vi "LQR_CLEst.vi"() -> ()   [LabVIEW 2019]
uses:
  <vilib>/Analysis/Matrix/Datatypes/RealMatrix.ctl
  <vilib>/Platform/TimedLoop/XDataNode/timing_clust.ctl
  <vilib>/Platform/TimedLoop/XDataNode/nitl_modes.ctl
  <vilib>/Platform/TimedLoop/XDataNode/wakeup.ctl
  <vilib>/Simulation/Shared/_Datatypes/SIM SISO Transfer Function.ctl
  <vilib>/myRIO/Instrument Drivers/Onboard IO/AI/typedefs/AI Reference.ctl
  <vilib>/myRIO/Common/Instrument Driver Framework/Utilities/typedefs/myRIO Generic Hardware Reference.ctl
  <vilib>/myRIO/Common/Instrument Driver Framework/Utilities/typedefs/Hardware Version Enum.ctl
  <vilib>/myRIO/Common/Instrument Driver Framework/Utilities/typedefs/myRIO v1.0 Reference.ctl
  <vilib>/myRIO/Common/Instrument Driver Framework/Utilities/typedefs/Generic FPGA Reference.ctl
  <vilib>/myRIO/Common/Instrument Driver Framework/myRIO v1.0/AI/typedefs/AI Channels List.ctl
  <vilib>/myRIO/Common/Instrument Driver Framework/myRIO v1.0/AI/typedefs/AI Channels Enum.ctl
  <vilib>/myRIO/Common/Instrument Driver Framework/Utilities/typedefs/Analog Scaling Constants List.ctl
  <vilib>/myRIO/Common/Instrument Driver Framework/Utilities/typedefs/Analog Scaling Constants.ctl
  <vilib>/userDefined/High Color/nirio_resource_hc.ctl
  <vilib>/myRIO/Instrument Drivers/Onboard IO/AO/typedefs/AO Reference.ctl
  <vilib>/myRIO/Common/Instrument Driver Framework/myRIO v1.0/AO/typedefs/AO Channels List.ctl
  <vilib>/myRIO/Common/Instrument Driver Framework/myRIO v1.0/AO/typedefs/AO Channels Enum.ctl
  <vilib>/myRIO/Common/Instrument Driver Framework/Utilities/vis/Is FPGA Ref Available.vi
  <vilib>/myRIO/Common/Instrument Driver Framework/myRIO v1.0/AI/vis/myRIO v1.1 Open AI.vi
  <vilib>/myRIO/Instrument Drivers/Onboard IO/AI/vis/Read.vi
  <vilib>/Simulation/DiscreteLinear/Implementation/NILVSim Discrete Transfer Function Direct.llb/SIM Discrete Transfer Function Diagram (SISO).vi
  <vilib>/myRIO/Common/Instrument Driver Framework/myRIO v1.0/AO/vis/myRIO v1.1 Open AO.vi
  <vilib>/myRIO/Instrument Drivers/Onboard IO/AO/vis/Write.vi
  <vilib>/myRIO/Common/Instrument Driver Framework/Utilities/vis/Validate Channels.vi
  <vilib>/myRIO/Common/Instrument Driver Framework/myRIO v1.0/AI/vis/myRIO v1.0 Reserve AI.vi
  <vilib>/Simulation/ContinuousLinear/Implementation/Shared/SIM Transfer Function Support.llb/SIM TransferFunction Normalize to Buffer.vi
  <vilib>/Simulation/DiscreteLinear/Implementation/Shared/SIM Init Discrete States.vi
  <vilib>/Simulation/DiscreteLinear/Implementation/NILVSim Discrete Transfer Function Direct.llb/SIM Transfer Function Direct core (SISO).vi
  <vilib>/myRIO/Common/Instrument Driver Framework/myRIO v1.0/AO/vis/myRIO v1.0 Reserve AO.vi
  <vilib>/myRIO/Common/Instrument Driver Framework/myRIO v1.0/AI/vis/myRIO v1.0 Build MUX Configuration AI.vi
  <vilib>/myRIO/Common/Instrument Driver Framework/myRIO v1.0/Resource Manager/vis/myRIO v1.0 Reserve Channel List.vi
  <vilib>/Simulation/ContinuousLinear/Implementation/Shared/SIM Transfer Function Support.llb/SIM TransferFunction Normalize.vi
  <vilib>/myRIO/Common/Instrument Driver Framework/myRIO v1.0/AO/vis/myRIO v1.0 Build MUX Configuration AO.vi
  <vilib>/myRIO/Common/Instrument Driver Framework/myRIO v1.0/Resource Manager/vis/myRIO v1.0 Reserve Channel.vi
  <vilib>/myRIO/Common/Instrument Driver Framework/myRIO v1.0/Resource Manager/vis/myRIO v1.0 Unreserve Channel.vi
  <vilib>/Simulation/Implementation/Shared/SIM Polynomials.llb/SIM Remove Zero Coefficients (DBL).vi
  <vilib>/myRIO/Common/Instrument Driver Framework/myRIO v1.0/Resource Manager/vis/myRIO v1.0 Build Mutex Name.vi
  <vilib>/Simulation/Implementation/Shared/SIM Polynomials.llb/SIM Divide Polynomials (DBL).vi
  <vilib>/Simulation/Implementation/Shared/SIM BuildSimErr.vi
  <vilib>/Utility/VariantDataType/GetNumericInfo.vi
  <vilib>/Utility/error.llb/Error Cluster From Error Code.vi
  <vilib>/myRIO/Common/Instrument Driver Framework/myRIO v1.0/myRIO v1.1 Open.vi
  <vilib>/myRIO/Common/Instrument Driver Framework/myRIO v1.0/AI/vis/myRIO v1.0 Get Scaling Constants AI.vi
  <vilib>/myRIO/Common/Instrument Driver Framework/Utilities/vis/IO Manager.vi
  <vilib>/myRIO/Common/Instrument Driver Framework/Utilities/vis/Configuration Manager.vi
  <vilib>/myRIO/Common/Instrument Driver Framework/myRIO v1.0/myRIO v1.0 Close.vi
  <vilib>/myRIO/Common/Instrument Driver Framework/myRIO v1.0/AI/vis/myRIO v1.0 Read AI.vi
  <vilib>/Analysis/Matrix/Numeric/Multiply/Multiply - RM,RM.vi
  <vilib>/Analysis/Matrix/Numeric/Subtract/Subtract (Elementwise) - R,RM.vi
  <vilib>/Analysis/Matrix/Numeric/Add/Add - RM,RM.vi
  <vilib>/myRIO/Common/Instrument Driver Framework/myRIO v1.0/AO/vis/myRIO v1.0 Get Scaling Constants AO.vi
  <vilib>/myRIO/Common/Instrument Driver Framework/myRIO v1.0/AO/vis/myRIO v1.0 Write AO.vi
  <vilib>/platform/TimedLoop/XDataNode/XDataNode.xnode
  <vilib>/Simulation/Implementation/XNodeFramework/SimXNode/SimX.xnode
  <vilib>/myRIO/Express VI/Onboard IO/AI/AI Express VI.xnode
  <vilib>/myRIO/Instrument Drivers/Onboard IO/AI/vis/myRIO AI Open.xnode
  <vilib>/myRIO/Express VI/Onboard IO/AO/AO Express VI.xnode
  <vilib>/myRIO/Instrument Drivers/Onboard IO/AO/vis/myRIO AO Open.xnode
  <vilib>/Analysis/Matrix/Numeric/Multiply/Multiply - RM,R.vi
  <vilib>/Platform/TimedLoop/XDataNode/XDNodeRunTimeDep.lvlib
  <vilib>/myRIO/Instrument Drivers/Onboard IO/AI/AI.lvlib
  <vilib>/myRIO/Instrument Drivers/Onboard IO/AO/AO.lvlib
  <vilib>/Analysis/Matrix/NI_Matrix.lvlib
panel:
  in  "amplitude":dbl=1.0 format="%0.2f"
  out "output y(k)":dbl=6.43996164946016e-05
  in  "D":dbl=7.3
  in  "P":dbl=5291.0
  out "x*y":dbl(graph)=-8.32082689025263
  in  "C":T1=[[1.0, 0.0]]
  out "transposed matrix":T1=[[7.6247197208905344e-06], [0.00010412510161981911]]
  in  "B":T1=[[0.0], [17.2685]]
  in  "A":T1=[[0.0, 1.0], [-5529.8, -0.5327]]
  in  "L":T1=[[2200.0], [1953300.0]]
  out "Iteration Duration":i64(graph)=347
  in  "esc":bool
  out "x[um]":cluster{dbl, dbl, dbl, dbl, "output y(k)":dbl}(graph)
  out "Current Output EM":dbl(graph)=0.03990822535355048
  in  "Stop EM + FRF":bool=TRUE
  out "left[V]":dbl=-0.0
  out "right[V]":dbl=-0.0
  out "um":dbl=376.9531636
  # "mA"
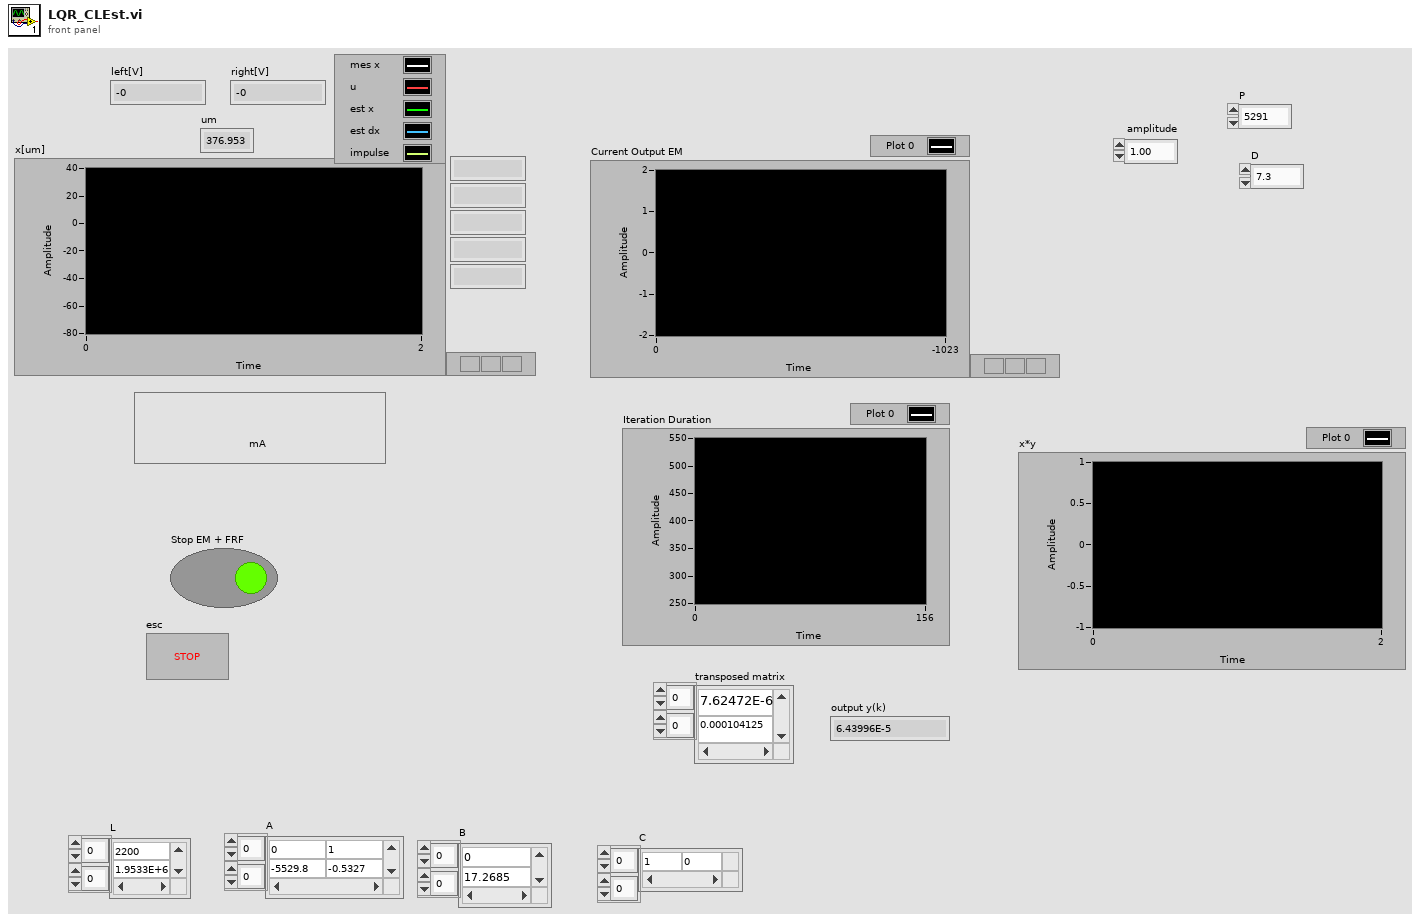
[diagram p1: front panel]
types:
  T1 = typedef "NI_Matrix.lvlib/RealMatrix.ctl" = dbl[][]
  T2 = typedef "XDNodeRunTimeDep.lvlib/timing_clust.ctl" = cluster{"Expected End [f-1]":u64, "Actual End [f-1]":u64, "Finished Late? [f-1]":bool, "Expected End [i-1]":u64, "Actual End [i-1]":u64, "Finished Late? [i-1]":bool, "Expected Start [i]":u64, "Actual Start [i]":u64, "Expected Start [f]":u64, "Actual Start [f]":u64, "Source Name":string, "Structure Name":string, "Period":i64, "Deadline":i64, "Offset":i64, "Start":i64, "Priority":i32, "Timeout":i32, "Mode":T3, "Wakeup Reason":T4, "Error":errorcluster, "Source Type":string, "Secondary Source Type":string, "Global End Time":u64, "Global Start Time":u64, "Frame Duration":u64, "Iteration Duration":u64, "Assigned CPU":i32, "I/O Scan Engine Mode":u32}
  T3 = typedef "XDNodeRunTimeDep.lvlib/nitl_modes.ctl" = enum32{"No Change", "Process missed periods, maintain original phase", "Discard missed periods, maintain original phase", "Process missed periods, ignore original phase", "Discard missed periods, ignore original phase"}
  T4 = typedef "XDNodeRunTimeDep.lvlib/wakeup.ctl" = enum32{"Normal", "Aborted", "Asynchronous wakeup", "Timing source error", "Timed loop error", "Timeout"}
  T5 = typedef "SIM SISO Transfer Function.ctl" = cluster{"Numerator":dbl[], "Denominator":dbl[]}
  T6 = typedef "AO.lvlib/AO Reference.ctl" = cluster{"myRIO Reference":T7, "AO Channel List":T11, "AO Scaling Constant List":T13}
  T7 = typedef "myRIO Generic Hardware Reference.ctl" = cluster{"myRIO Model":T8, "myRIO Hardware Reference":T9}
  T8 = typedef "Hardware Version Enum.ctl" = enum16{"Unknown", "myRIO-1900", "myRIO-1950", "roboRIO", "NI ELVIS RIO CM", "ELVIS III"}
  T9 = typedef "myRIO v1.0 Reference.ctl" = cluster{"Generic FPGA Reference":T10, "Allow multiple opens":bool}
  T10 = typedef "Generic FPGA Reference.ctl" = refnum<k20>
  T11 = typedef "AO Channels List.ctl" = T12[]
  T12 = typedef "AO Channels Enum.ctl" = enum16{"Not Connected", "AudioOut/Left", "AudioOut/Right", "C/AO0", "C/AO1", "A/AO0", "A/AO1", "B/AO0", "B/AO1"}
  T13 = typedef "Analog Scaling Constants List.ctl" = T14[]
  T14 = typedef "Analog Scaling Constants.ctl" = cluster{"LSB Weight (Volts)":dbl, "Offset (Volts)":dbl, "Signed?":bool}
  T15 = typedef "nirio_resource_hc.ctl" = tag
  T16 = typedef "AI.lvlib/AI Reference.ctl" = cluster{"myRIO Reference":T7, "AI Channels List":T17, "AI Scaling Constants List":T13}
  T17 = typedef "AI Channels List.ctl" = T18[]
  T18 = typedef "AI Channels Enum.ctl" = enum16{"Not Connected", "AudioIn/Left", "AudioIn/Right", "C/AI0", "C/AI1", "A/AI0", "A/AI1", "A/AI2", "A/AI3", "A/AI4", "A/AI5", "A/AI6", "A/AI7", "B/AI0", "B/AI1", "B/AI2", "B/AI3", "B/AI4", "B/AI5", "B/AI6", "B/AI7", "AI/AI0", "AI/AI1", "AI/AI2", "AI/AI3", "A/AI0 (DIFF)", "A/AI1 (DIFF)", "A/AI2 (DIFF)", "A/AI3 (DIFF)", "B/AI0 (DIFF)", "B/AI1 (DIFF)", "B/AI2 (DIFF)", "B/AI3 (DIFF)"}
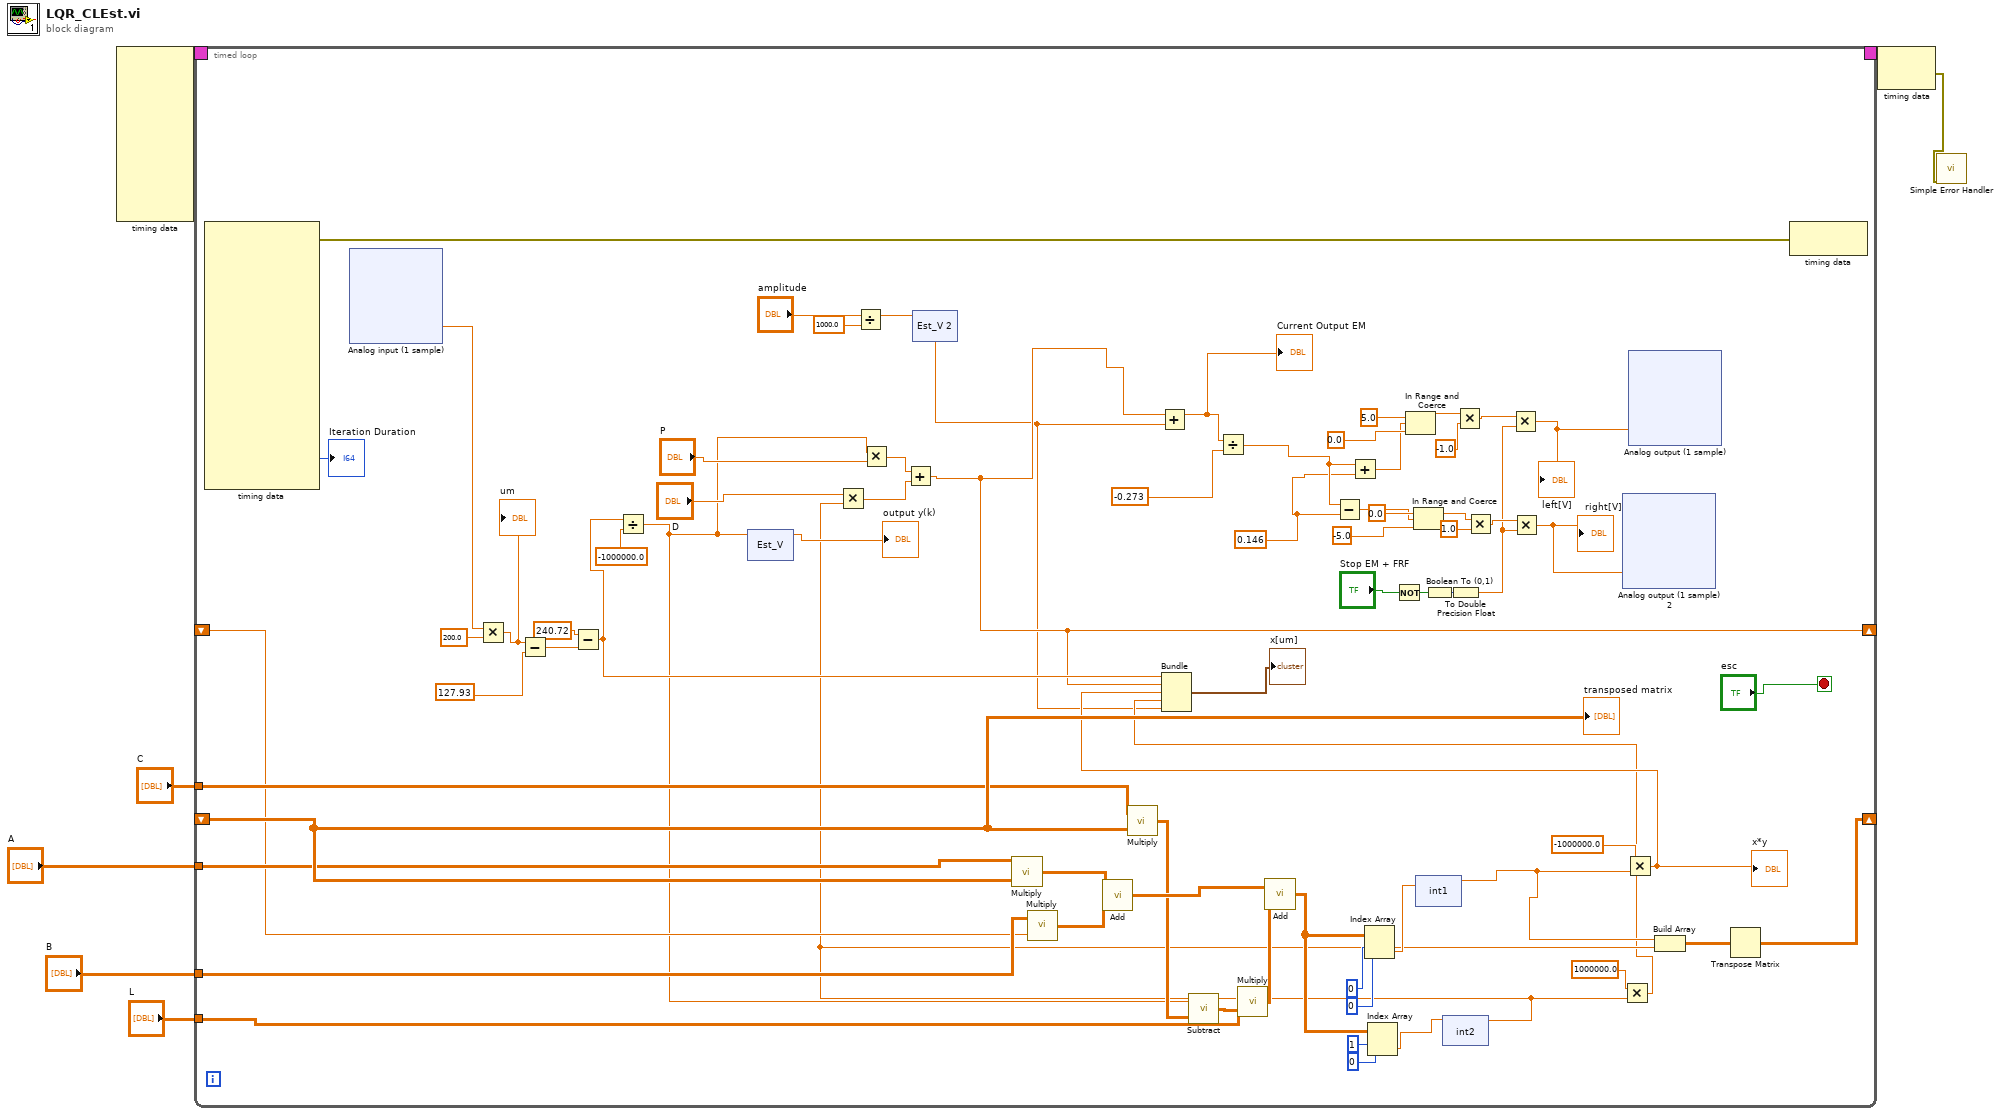
[diagram p0: block diagram]
diagram:
  n1 = node-c288() -> (w7:T2)  [unwired: 10 in]
  n2 = timed-loop {
    timing: w7 -> [_]
    timing-out: [_] -> w6
    shift-right: [w34] -> _
    shift-left: _ -> [w35]
    tunnel: "A" -> [w31]
    tunnel: "B" -> [w30]
    tunnel: "C" -> [w29]
    tunnel: "L" -> [w28]
    shift-right: [w9] -> _
    shift-left: _ -> [w25]
    stop <- "esc" stop-if-true
    w57 = 0.146 ("y")
    n3 = node-c288() -> (w79:errorcluster, →"Iteration Duration":i64)  [unwired: 1 in, 15 out]
    n4 = xnode "Analog input (1 sample)"() -> ("C/AI1 (AI1)"=w53:dbl)  [unwired: 1 in, 1 out]
    n5 = Multiply(x=w53, y=200.0) -> (x*y=w77:dbl)
    "um" <- w77
    n6 = Subtract(x=w77, y=127.93) -> (x-y=w76:dbl)
    n7 = Subtract(x=240.72, y=w76) -> (x-y=w47:dbl)
    n8 = Divide(x=w47, y=-1000000.0) -> (x/y=w18:dbl)
    n9 = xnode "Est_V"("input u(k)"=w18) -> ("output y(k)"=→"output y(k)":dbl)  [unwired: 2 in, 1 out]
    n10 = Divide(x="amplitude", y=1000.0) -> (x/y=w16:dbl)
    n11 = Multiply(x=w18, y="P") -> (x*y=w27:dbl)
    n12 = xnode "Est_V 2"("input u(k)"=w16) -> ("output y(k)"=w8:dbl)  [unwired: 2 in, 1 out]
    n13 = call-poly <vilib>:"Multiply.vi"("Real Matrix B"=w35, "Real Matrix A"=w31) -> ("A * B"=w46:T1)
    n14 = call-poly <vilib>:"Multiply.vi"("Real Scalar c"=w25, "Real Matrix A"=w30) -> ("A * c"=w45:T1)
    n15 = call-poly <vilib>:"Add.vi"("Real Matrix B"=w45, "Real Matrix A"=w46) -> ("A + B"=w44:T1)
    n16 = call-poly <vilib>:"Multiply.vi"("Real Matrix B"=w35, "Real Matrix A"=w29) -> ("A * B"=w33:T1)
    n17 = call-poly <vilib>:"Subtract.vi"("Real Matrix A"=w33, "Real Scalar c"=w18) -> ("c - A"=w37:T1)
    n18 = call-poly <vilib>:"Multiply.vi"("Real Matrix B"=w37, "Real Matrix A"=w28) -> ("A * B"=w43:T1)
    n19 = call-poly <vilib>:"Add.vi"("Real Matrix B"=w43, "Real Matrix A"=w44) -> ("A + B"=w38:T1)
    n20 = Index Array(array=w38, index (row)=0, index (col)=0 ("disabled index (col)")) -> (element=w22:dbl)
    n21 = Index Array(array=w38, index (row)=1, index (col)=0 ("disabled index (col)")) -> (element=w21:dbl)
    n22 = Not(x="Stop EM + FRF") -> (.not. x?=w64:bool)
    n23 = xnode "int1"("input u(k)"=w22) -> ("output y(k)"=w19:dbl)  [unwired: 2 in, 1 out]
    n24 = Boolean To (0,1)(Boolean=w64) -> (0, 1=w66:i16)
    n25 = xnode "int2"("input u(k)"=w21) -> ("output y(k)"=w12:dbl)  [unwired: 2 in, 1 out]
    n26 = Multiply(x="D", y=w12) -> (x*y=w26:dbl)
    n27 = Add(x=w27, y=w26) -> (x+y=w9:dbl)
    n28 = Add(x=w9, y=w8) -> (x+y=w14:dbl)
    "Current Output EM" <- w14
    n29 = Divide(x=w14, y=-0.273) -> (x/y=w58:dbl)
    n30 = Subtract(x=w58, y=w57) -> (x-y=w59:dbl)
    n31 = Add(x=w58, y=w57) -> (x+y=w60:dbl)
    n32 = In Range and Coerce(upper limit=5.0 ("x"), x=w60, lower limit=0.0) -> (coerced(x)=w50:dbl)  [unwired: 1 out]
    n33 = In Range and Coerce(upper limit=0.0 ("x"), x=w59, lower limit=-5.0) -> (coerced(x)=w69:dbl)  [unwired: 1 out]
    n34 = To Double Precision Float(number=w66) -> (double precision float=w54:dbl)
    n35 = Multiply(x=w50, y=-1.0) -> (x*y=w56:dbl)
    n36 = Multiply(x=w69, y=1.0) -> (x*y=w55:dbl)
    n37 = Multiply(x=w56, y=w54) -> (x*y=w52:dbl)
    "left[V]" <- w52
    n38 = Multiply(x=w55, y=w54) -> (x*y=w51:dbl)
    "right[V]" <- w51
    n39 = Multiply ("Multiply.vi")(x=1000000.0 ("y"), y=w12) -> (x*y=w10:dbl)
    n40 = xnode "Analog output (1 sample) 2"("C/AO1 (AO1)"=w51) -> ()  [unwired: 1 in, 1 out]
    n41 = Multiply ("Multiply.vi")(x=-1000000.0 ("y"), y=w19) -> (x*y=w11:dbl)
    "x*y" <- w11
    n42 = Bundle(w47, w9, w11, w10, "output y(k)"=w8) -> (→"x[um]":cluster{dbl, dbl, dbl, dbl, "output y(k)":dbl})  [unwired: 1 in]
    n43 = xnode "Analog output (1 sample)"("C/AO0 (AO0)"=w52) -> ()  [unwired: 1 in, 1 out]
    n44 = Build Array(w19, w12) -> (w36:T1)
    n45 = Transpose Matrix(1:w36) -> (0:w34:T1)
    n46 = node-c288(w79) -> ()  [unwired: 1 out]
    "transposed matrix" <- w35
  }
  n47 = node-c288(w6) -> (w5:errorcluster)
  n48 = call <vilib>:"Simple Error Handler.vi"("error in (no error)"=w5) -> ()  [unwired: 4 in, 5 out]
